vi "Prog_Revision_Date.vi"(5 "Input string":string) -> (0 "Revision time (s)":u32, 2 "svnBaseRevision":u32, 3 "Prog's last revision date":string)   [LabVIEW 2012]
uses:
  <vilib>/Utility/miscctls.llb/LVDateTimeRec.ctl
panel:
  out "source":string
  out "Prog's last revision time":string
  out "RevisionData":string
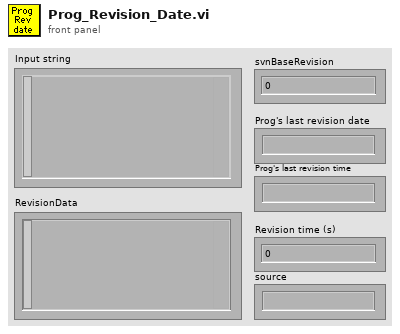
[diagram p1: front panel]
types:
  T1 = typedef "LVDateTimeRec.ctl" = cluster{"fractional second":dbl, "second":i32, "minute":i32, "hour":i32, "day of month":i32, "month":i32, "year":i32, "day of week":i32, "day of year":i32, "DST":i32}
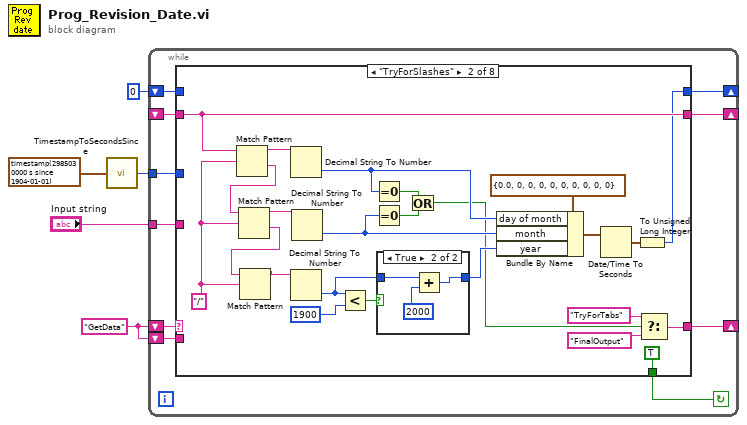
[diagram p0: block diagram]
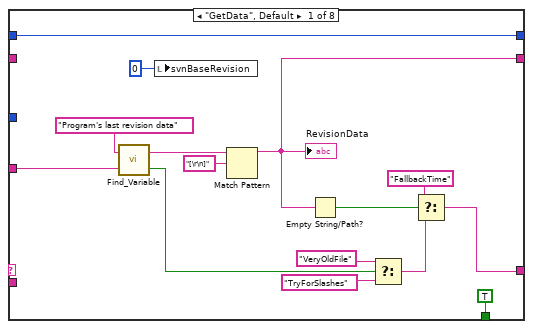
[diagram p2: hidden frame]
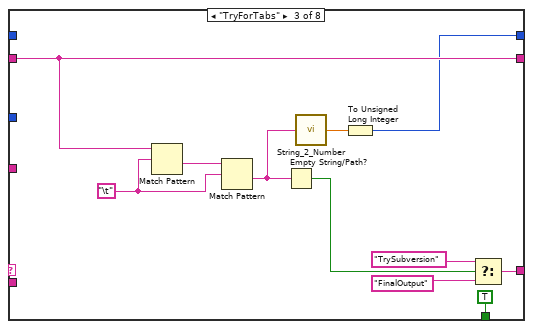
[diagram p4: hidden frame]
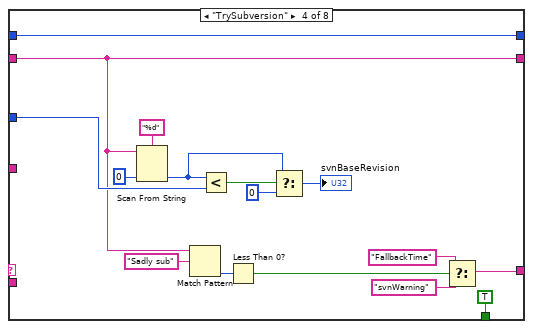
[diagram p5: hidden frame]
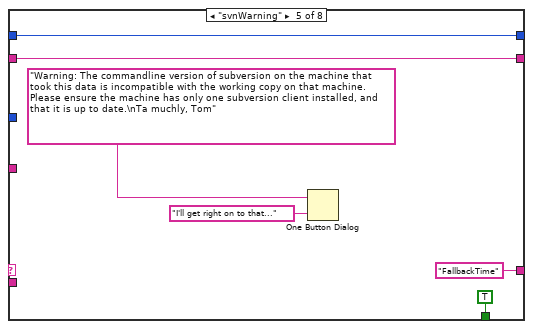
[diagram p6: hidden frame]
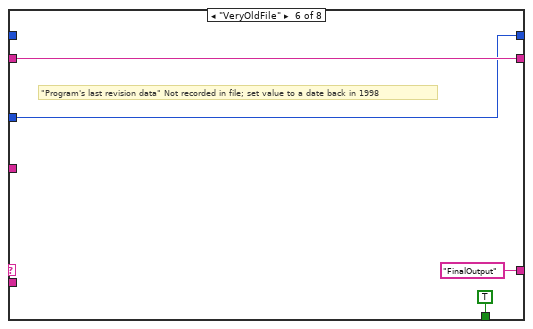
[diagram p7: hidden frame]
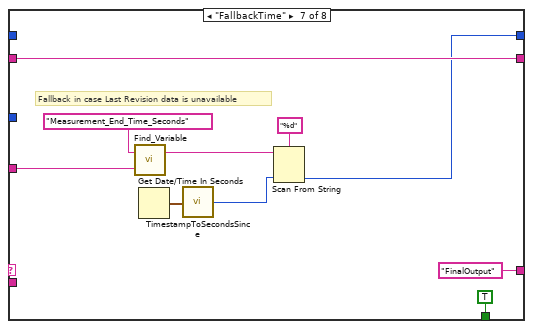
[diagram p8: hidden frame]
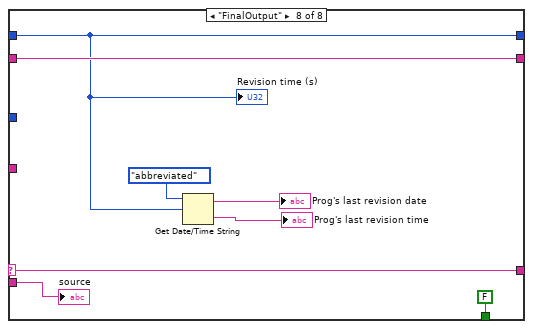
[diagram p9: hidden frame]
diagram:
  w1 = "GetData"
  n1 = call "TimestampToSecondsSince.vi"("Time Stamp Control"=timestamp(2985030000 s since 1904-01-01)) -> ("unsigned 32bit integer"=w2:u32)
  n2 = while {
    tunnel: "Input string" -> [w15]
    shift-right: [w13] -> _
    shift-left: w1 -> [w14]
    shift-right: [w12] -> _
    shift-left: u32 0 -> [w11]
    shift-right: [w9] -> _
    shift-left: _ -> [w8]
    tunnel: w2 -> [w7]
    shift-left: w1 -> [w6]
    stop <- w10 continue-if-true
    n3 = case shown="\"TryForSlashes\"" w14 {
      selector: w14 -> [_ _ _ _ _ _ _ w107]
      tunnel: w15 -> [w27 _ _ _ _ _ w101 _]
      tunnel: [w18 w38 w66 w73 "FallbackTime" ("t") "FinalOutput" "FinalOutput" w107] -> w13
      tunnel: [w24 w40 w60 w85 w91 w92 w98 w109] -> w12
      tunnel: w11 -> [w24 _ _ w85 w91 _ _ w109]
      tunnel: [TRUE TRUE TRUE TRUE TRUE TRUE TRUE FALSE] -> w10
      tunnel: [w21 w41 w67 w76 w90 w93 w105 w113] -> w9
      tunnel: w8 -> [_ w41 w67 w76 w90 w93 w105 w113]
      tunnel: w7 -> [_ _ _ w82 _ w92 _ _]
      tunnel: w6 -> [_ _ _ _ _ _ _ w106]
      frame "GetData", Default {
        n4 = call "Find_Variable.vi"("Input string"=w27, "Variable name"="Program's last revision data") -> ("No Match?"=w26:bool, "After  Matched string"=w29:string)
        n5 = local write "svnBaseRevision"(0 ("svnBaseRevision")) -> ()
        n6 = Match Pattern(string=w29, regular expression="[\r\n]") -> (before substring=w21:string)  [unwired: 4 out]
        "RevisionData" <- w21
        n7 = Empty String/Path?(string/path=w21) -> (empty?=w19:bool)
        n8 = Select(t="VeryOldFile", s=w26, f="TryForSlashes") -> (s? t:f=w20:string)
        n9 = Select(t="FallbackTime", s=w19, f=w20) -> (s? t:f=w18:string)
      }
      frame "TryForSlashes" {
        w42 = "/" ("search char (-)")
        n10 = Match Pattern(string=w41, regular expression=w42) -> (before substring=w43:string, after substring=w44:string)  [unwired: 3 out]
        n11 = Match Pattern(string=w44, regular expression=w42) -> (before substring=w45:string, after substring=w47:string)  [unwired: 3 out]
        n12 = Match Pattern(string=w47, regular expression=w42) -> (before substring=w46:string)  [unwired: 4 out]
        n13 = Decimal String To Number(string=w43) -> (number=w35:i32)  [unwired: 3 out]
        n14 = Decimal String To Number(string=w46) -> (number=w51:i32)  [unwired: 3 out]
        n15 = Decimal String To Number(string=w45) -> (number=w34:i32)  [unwired: 3 out]
        n16 = Less?(x=w51, y=1900) -> (x < y?=w50:bool)
        n17 = Equal To 0?(x=w35) -> (x = 0?=w33:bool)
        n18 = Equal To 0?(x=w34) -> (x = 0?=w32:bool)
        n19 = case shown="True" w50 {
          tunnel: w51 -> [w55 w57]
          tunnel: [w55 w56] -> w52
          frame False {
          }
          frame True {
            n20 = Add(x=w57, y=2000) -> (x+y=w56:i32)
          }
        }
        n21 = Or(x=w33, y=w32) -> (x .or. y?=w31:bool)
        n22 = Bundle By Name(cluster=T1 {"fractional second"=0.0, "second"=0, "minute"=0, "hour"=0, "day of month"=0, "month"=0, "year"=0, "day of week"=0, "day of year"=0, "DST"=0} ("date time rec"), "day of month"=w35, "month"=w34, "year"=w52) -> (w54:T1)
        n23 = Date/Time To Seconds(2:w54) -> (0:w48:timestamp)  [unwired: 1 in]
        n24 = To Unsigned Long Integer(number=w48) -> (unsigned 32bit integer=w40:u32)
        n25 = Select(t="TryForTabs", s=w31, f="FinalOutput") -> (s? t:f=w38:string)
      }
      frame "TryForTabs" {
        w69 = "\t"
        n26 = Match Pattern(string=w67, regular expression=w69) -> (after substring=w68:string)  [unwired: 4 out]
        n27 = Match Pattern(string=w68, regular expression=w69) -> (after substring=w61:string)  [unwired: 4 out]
        n28 = Empty String/Path?(string/path=w61) -> (empty?=w65:bool)
        n29 = call "String_2_Number.vi"("Value"=w61) -> ("Numeric"=w62:dbl)
        n30 = To Unsigned Long Integer(number=w62) -> (unsigned 32bit integer=w60:u32)
        n31 = Select(t="TrySubversion", s=w65, f="FinalOutput") -> (s? t:f=w66:string)
      }
      frame "TrySubversion" {
        n32 = Scan From String(format string="%d", input string=w76, default 1=u32 0 ("unsigned 32bit integer")) -> (output 1=w80:u32)  [unwired: 2 in, 3 out]
        n33 = Match Pattern(string=w76, regular expression="Sadly sub") -> (offset past match=w74:i32)  [unwired: 1 in, 3 out]
        n34 = Less?(x=w80, y=w82) -> (x < y?=w81:bool)
        n35 = Less Than 0?(x=w74) -> (x < 0?=w71:bool)
        n36 = Select(t=w80, s=w81, f=u32 0) -> (s? t:f=→"svnBaseRevision":u32)
        n37 = Select(t="FallbackTime", s=w71, f="svnWarning" ("t")) -> (s? t:f=w73:string)
      }
      frame "svnWarning" {
        n38 = One Button Dialog(message="Warning: The commandline version of subversion on the machine that took this data is incompatible with the working copy on that machine. Please ensure the machine has only one subversion client installed, and that it is up to date.\nTa muchly, Tom", button name ("OK")="I'll get right on to that...") -> ()  [unwired: 1 out]
      }
      frame "VeryOldFile" {
        # "\"Program's last revision data\" Not recorded in file; set value to a date back in 1998"
      }
      frame "FallbackTime" {
        # "Fallback in case Last Revision data is unavailable"
        n39 = call "Find_Variable.vi"("Input string"=w101, "Variable name"="Measurement_End_Time_Seconds") -> ("After  Matched string"=w102:string)  [unwired: 1 out]
        n40 = Get Date/Time In Seconds() -> (seconds since 1Jan1904=w97:timestamp)
        n41 = call "TimestampToSecondsSince.vi"("Time Stamp Control"=w97) -> ("unsigned 32bit integer"=w96:u32)
        n42 = Scan From String(format string="%d", input string=w102, default 1=w96) -> (output 1=w98:u32)  [unwired: 2 in, 3 out]
      }
      frame "FinalOutput" {
        n43 = Get Date/Time String(date format (0)=enum16{"short", "long", "abbreviated"}."abbreviated", seconds (now)=w109) -> (date string=→"Prog's last revision date":string, time string=→"Prog's last revision time":string)  [unwired: 1 out]
        "Revision time (s)" <- w109
        "source" <- w106
      }
    }
  }
